vi "start_stream_only.vi"(6 "Period [ms]":i32=500 min=1 max=60000, 8 "error in (no error)":errorcluster, 10 "Scan Rate (Hz)":dbl=250.0 format="%.3f", 11 "Handle In":i32) -> (0 "error out":errorcluster, 1 "NumReadAddresses":i32, 2 "ScansPerRead Out":i32, 3 "Handle Out":i32)   [LabVIEW 2025, in "LabJackEKG.lvlib"]
uses:
  LabJackEKG.lvlib
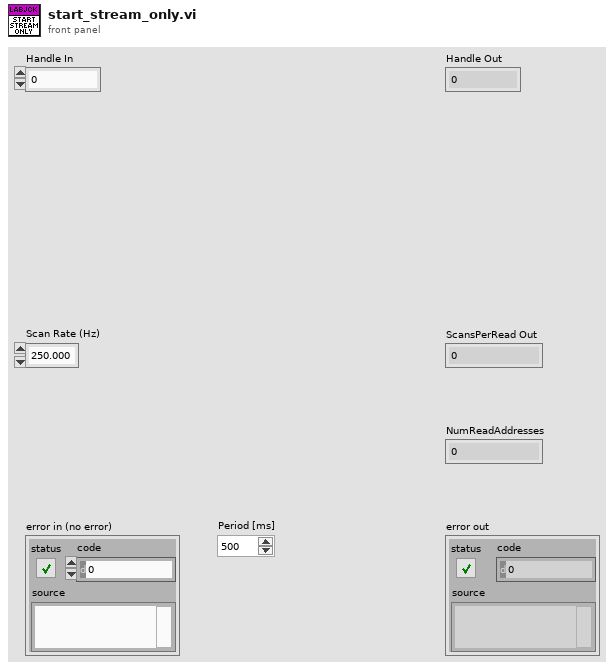
[diagram p1: front panel]
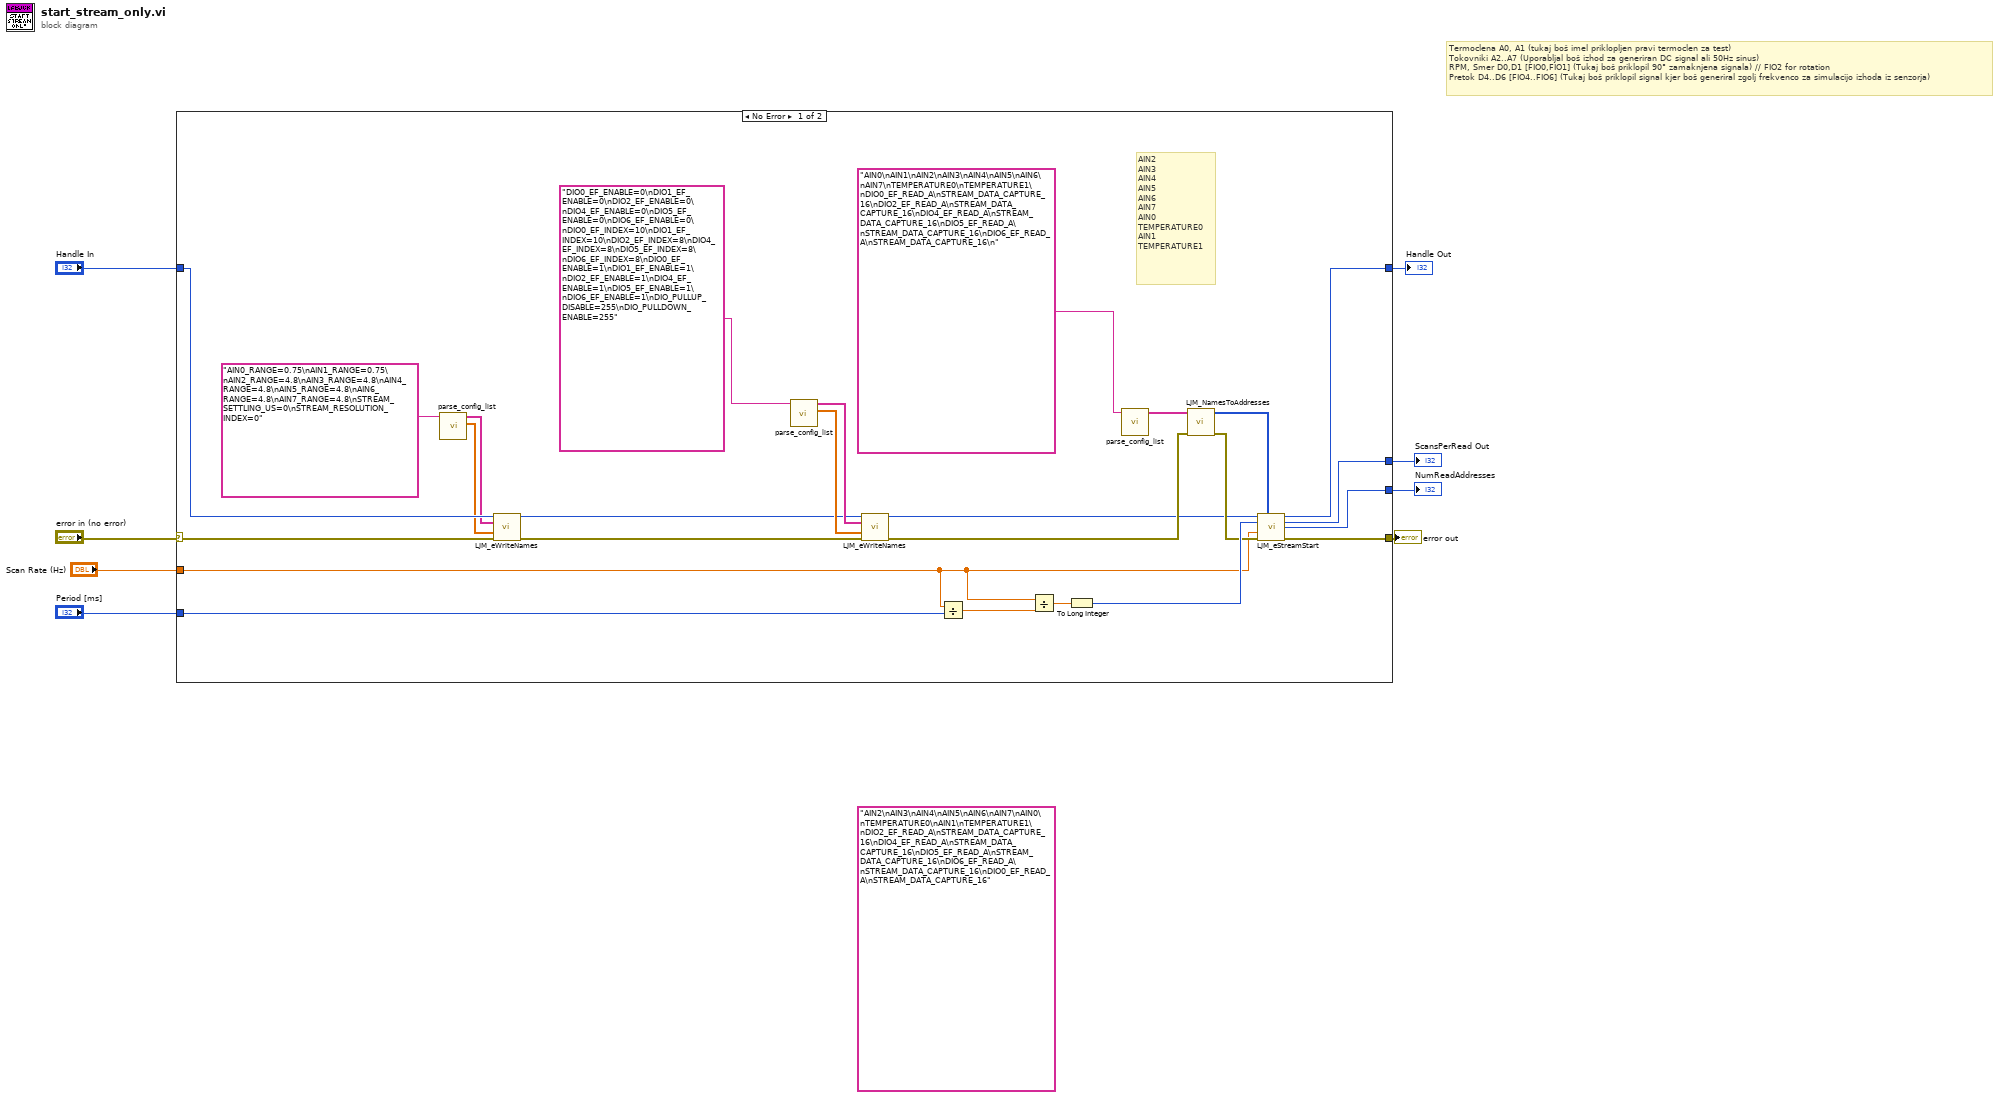
[diagram p0: block diagram]
diagram:
  (unwired) "AIN2\nAIN3\nAIN4\nAIN5\nAIN6\nAIN7\nAIN0\nTEMPERATURE0\nAIN1\nTEMPERATURE1\nDIO2_EF_READ_A\nSTREAM_DATA_CAPTURE_16\nDIO4_EF_READ_A\nSTREAM_DATA_CAPTURE_16\nDIO5_EF_READ_A\nSTREAM_DATA_CAPTURE_16\nDIO6_EF_READ_A\nSTREAM_DATA_CAPTURE_16\nDIO0_EF_READ_A\nSTREAM_DATA_CAPTURE_16" ("String")
  # "Termoclena A0, A1 (tukaj boš imel priklopljen pravi termoclen za test)\nTokovniki A2..A7 (Uporabljal boš izhod za generiran DC signal ali 50Hz sinus)\nRPM, Smer D0,D1 [FIO0,FIO1] (Tukaj boš priklopil 90° zamaknjena signala) // FIO2 for rotation\nPretok D4..D6 [FIO4..FIO6] (Tukaj boš priklopil signal kjer boš generiral zgolj frekvenco za simulacijo izhoda iz senzorja)"
  n1 = case shown="No Error" "error in (no error)" {
    selector: "error in (no error)" -> [w33 w35]
    tunnel: [w29 w34] -> w8
    tunnel: "Handle In" -> [w32 w34]
    tunnel: [w30 w35] -> w5
    tunnel: [w27 _] -> w4
    tunnel: [w26 _] -> w3
    tunnel: "Period [ms]" -> [w25 _]
    tunnel: "Scan Rate (Hz)" -> [w10 _]
    frame No Error {
      # "AIN2\nAIN3\nAIN4\nAIN5\nAIN6\nAIN7\nAIN0\nTEMPERATURE0\nAIN1\nTEMPERATURE1"
      n2 = call "parse_config_list.vi"("String"="AIN0_RANGE=0.75\nAIN1_RANGE=0.75\nAIN2_RANGE=4.8\nAIN3_RANGE=4.8\nAIN4_RANGE=4.8\nAIN5_RANGE=4.8\nAIN6_RANGE=4.8\nAIN7_RANGE=4.8\nSTREAM_SETTLING_US=0\nSTREAM_RESOLUTION_INDEX=0") -> ("Values"=w21:dbl[], "Names"=w22:string[])  [unwired: 9 in]
      n3 = call <vilib>:"LJM_eWriteNames.vi"("Handle In"=w32, "aNames"=w22, "aValuesIn"=w21, "error in"=w33) -> ("Handle Out"=w12:i32, "error out"=w13:errorcluster)  [unwired: 9 in, 1 out]
      n4 = call "parse_config_list.vi"("String"="DIO0_EF_ENABLE=0\nDIO1_EF_ENABLE=0\nDIO2_EF_ENABLE=0\nDIO4_EF_ENABLE=0\nDIO5_EF_ENABLE=0\nDIO6_EF_ENABLE=0\nDIO0_EF_INDEX=10\nDIO1_EF_INDEX=10\nDIO2_EF_INDEX=8\nDIO4_EF_INDEX=8\nDIO5_EF_INDEX=8\nDIO6_EF_INDEX=8\nDIO0_EF_ENABLE=1\nDIO1_EF_ENABLE=1\nDIO2_EF_ENABLE=1\nDIO4_EF_ENABLE=1\nDIO5_EF_ENABLE=1\nDIO6_EF_ENABLE=1\nDIO_PULLUP_DISABLE=255\nDIO_PULLDOWN_ENABLE=255") -> ("Values"=w16:dbl[], "Names"=w15:string[])  [unwired: 9 in]
      n5 = call <vilib>:"LJM_eWriteNames.vi"("Handle In"=w12, "aNames"=w15, "aValuesIn"=w16, "error in"=w13) -> ("Handle Out"=w11:i32, "error out"=w14:errorcluster)  [unwired: 9 in, 1 out]
      n6 = Divide(x=w10, y=w25) -> (x/y=w24:dbl)
      n7 = Divide(x=w10, y=w24) -> (x/y=w31:dbl)
      n8 = To Long Integer(number=w31) -> (32bit integer=w28:i32)
      n9 = call "parse_config_list.vi"("String"="AIN0\nAIN1\nAIN2\nAIN3\nAIN4\nAIN5\nAIN6\nAIN7\nTEMPERATURE0\nTEMPERATURE1\nDIO0_EF_READ_A\nSTREAM_DATA_CAPTURE_16\nDIO2_EF_READ_A\nSTREAM_DATA_CAPTURE_16\nDIO4_EF_READ_A\nSTREAM_DATA_CAPTURE_16\nDIO5_EF_READ_A\nSTREAM_DATA_CAPTURE_16\nDIO6_EF_READ_A\nSTREAM_DATA_CAPTURE_16\n") -> ("Names"=w19:string[])  [unwired: 9 in, 1 out]
      n10 = call <vilib>:"LJM_NamesToAddresses.vi"("error in"=w14, "aNames"=w19) -> ("error out"=w17:errorcluster, "aAddresses"=w18:i32[])  [unwired: 7 in, 1 out]
      n11 = call <vilib>:"LJM_eStreamStart.vi"("Handle In"=w11, "aScanList"=w18, "ScansPerRead"=w28, "ScanRate"=w10, "error in"=w17) -> ("Handle Out"=w29:i32, "ScansPerRead Out"=w26:i32, "NumReadAddresses"=w27:i32, "error out"=w30:errorcluster)  [unwired: 5 in, 2 out]
    }
    frame Error {
    }
  }
  "error out" <- w5
  "Handle Out" <- w8
  "ScansPerRead Out" <- w3
  "NumReadAddresses" <- w4
